vi "Publish Client Updates.vi"(8 "error in (no error)":errorcluster, 10 "Client Info Loop Data":T1, 11 "TCPMessaging in":refnum<class "TCPMessaging.lvclass">) -> (0 "error out":errorcluster, 3 "TCPMessaging out":refnum<class "TCPMessaging.lvclass">)   [LabVIEW 2020, in "Vecto.lvlib" / "TCPMessaging.lvclass"]
uses:
  TCPMessaging.lvclass
  Client Info Loop Data.ctl
  Connected Client.ctl
  Client Info.ctl
  proto/TcpClientInfo/Data.ctl
  proto/TcpClientList/Data.ctl
  TCPMessaging.lvclass/TCPMessaging.ctl
  proto/TcpClientInfo/TcpClientInfo.lvlib
  proto/TcpClientList/TcpClientList.lvlib
  TCPMessageService/TCPMessageAPI.lvclass
  VectoConfig/VectoConfig.lvlib
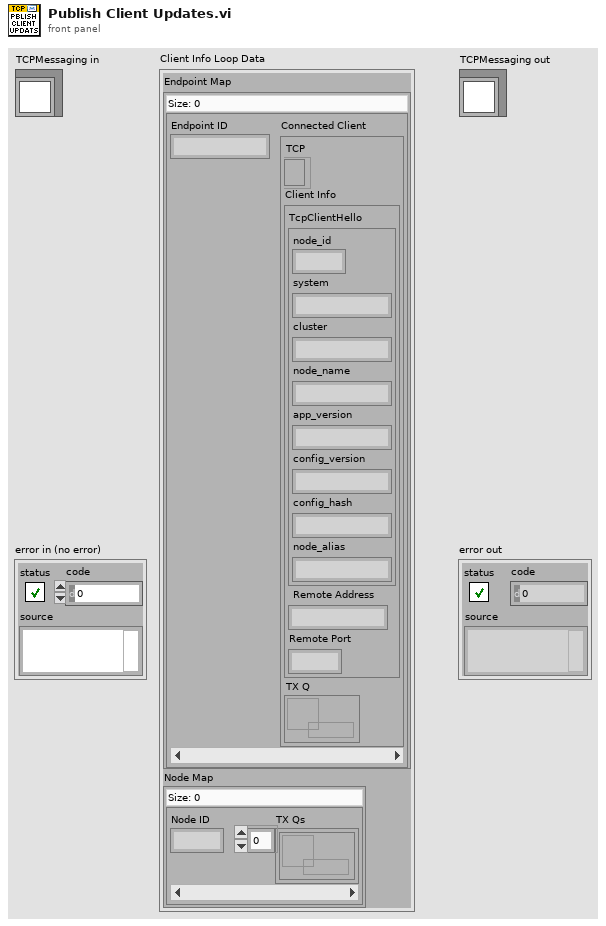
[diagram p1: front panel]
types:
  T1 = typedef "Vecto.lvlib/TCPMessaging.lvclass/Client Info Loop Data.ctl" = cluster{"Endpoint Map":map{string, T2}, "Node Map":map{u32, refnum<queue>[]}}
  T2 = typedef "Vecto.lvlib/TCPMessaging.lvclass/Connected Client.ctl" = cluster{"TCP":refnum<k5>, "Client Info":T3, "TX Q":refnum<queue>}
  T3 = typedef "VectoConfig.lvlib/Client Info.ctl" = cluster{"TcpClientHello":cluster{"node_id":u32, "system":string, "cluster":string, "node_name":string, "app_version":string, "config_version":string, "config_hash":string, "node_alias":string}, "Remote Address":string, "Remote Port":u16}
  T4 = typedef "TcpClientList.lvlib/Data.ctl" = cluster{"clients":T5[]}
  T5 = typedef "TcpClientInfo.lvlib/Data.ctl" = cluster{"node_id":u32, "node_name":string, "app_version":string, "config_version":string, "config_hash":string, "node_alias":string, "address":string}
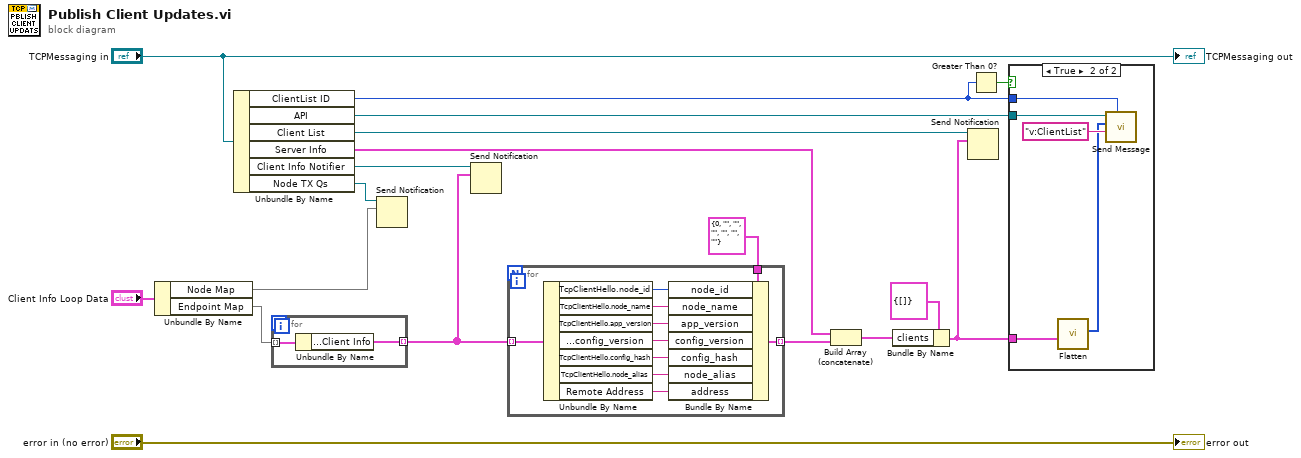
[diagram p0: block diagram]
diagram:
  n1 = Unbundle By Name("Client Info Loop Data") -> ("Node Map"=w12:map{u32, refnum<queue>[]}, "Endpoint Map"=w16:map{string, T2})
  n2 = Unbundle By Name("TCPMessaging in") -> ("ClientList ID"=w10:u32, "API"=w11:refnum<class "TCPMessageAPI.lvclass">, "Client List"=w7:refnum<notifier>, "Server Info"=w2:T5, "Client Info Notifier"=w14:refnum<notifier>, "Node TX Qs"=w15:refnum<notifier>)
  n3 = for {
    tunnel: w16 -> [w20] mode=indexing
    tunnel: [w19] -> w1 mode=indexing
    n4 = Unbundle By Name(w20) -> ("Connected Client.Client Info"=w19:T3)
  }
  n5 = Send Notification(notification=w12, notifier=w15) -> ()  [unwired: 1 in, 2 out]
  n6 = Send Notification(notification=w1, notifier=w14) -> ()  [unwired: 1 in, 2 out]
  n7 = for {
    tunnel: w1 -> [w29] mode=indexing
    tunnel: [w30] -> w5 mode=indexing
    tunnel: T5 {"node_id"=0, "node_name"="", "app_version"="", "config_version"="", "config_hash"="", "node_alias"="", "address"=""} ("TcpClientInfo") -> [w21]
    n8 = Unbundle By Name(w29) -> ("TcpClientHello.node_id"=w28:u32, "TcpClientHello.node_name"=w27:string, "TcpClientHello.app_version"=w26:string, "TcpClientHello.config_version"=w25:string, "TcpClientHello.config_hash"=w24:string, "TcpClientHello.node_alias"=w23:string, "Remote Address"=w22:string)
    n9 = Bundle By Name(cluster=w21, "node_id"=w28, "node_name"=w27, "app_version"=w26, "config_version"=w25, "config_hash"=w24, "node_alias"=w23, "address"=w22) -> (w30:T5)
  }
  n10 = Build Array (concatenate)(w2, w5) -> (w3:T5[])
  n11 = Bundle By Name(cluster=T4 {"clients"=[]} ("TcpClientList"), "clients"=w3) -> (w4:T4)
  n12 = Send Notification(notification=w4, notifier=w7) -> ()  [unwired: 1 in, 2 out]
  n13 = Greater Than 0?(x=w10) -> (x > 0?=w9:bool)
  n14 = case shown="True" w9 {
    tunnel: w11 -> [_ w35]
    tunnel: w10 -> [_ w32]
    tunnel: w4 -> [_ w31]
    frame False {
      # "Client list target group not configured, don't bother serializing and publishing."
    }
    frame True {
      n15 = call "Flatten.vi"("Data"=w31) -> ("Buffer"=w33:u8[])  [unwired: 9 in, 1 out]
      n16 = call "Send Message.vi"("Target ID"=w32, "Type"="v:ClientList", "Payload"=w33, "TCPMessageService in"=w35) -> ()  [unwired: 6 in, 2 out]
    }
  }
  "error out" <- "error in (no error)"
  "TCPMessaging out" <- "TCPMessaging in"
